vi "HalfLatch.vi"(11 "Input":bool) -> (3 "Output":bool)   [LabVIEW 2012]
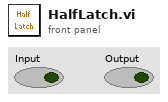
[diagram p1: front panel]
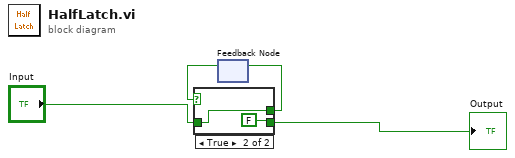
[diagram p0: block diagram]
diagram:
  n1 = feedback #1() -> (w3:bool)  [unwired: 1 in]
  n2 = case shown="True" w3 {
    tunnel: "Input" -> [w5 w7]
    tunnel: [w5 w7] -> w2
    tunnel: [w5 FALSE] -> w4
    frame False {
    }
    frame True {
    }
  }
  "Output" <- w4
  n3 = feedback-in #1(w2) -> ()
